vi "Error Handler.vi"(8 "error in (no error)":errorcluster) -> (0 "error out (no error)":errorcluster)   [LabVIEW 2019]
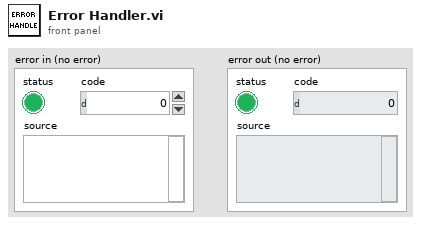
[diagram p1: front panel]
types:
  T1 = enum16{"open", "replace", "create", "open or create", "replace or create", "replace or create with confirmation"}
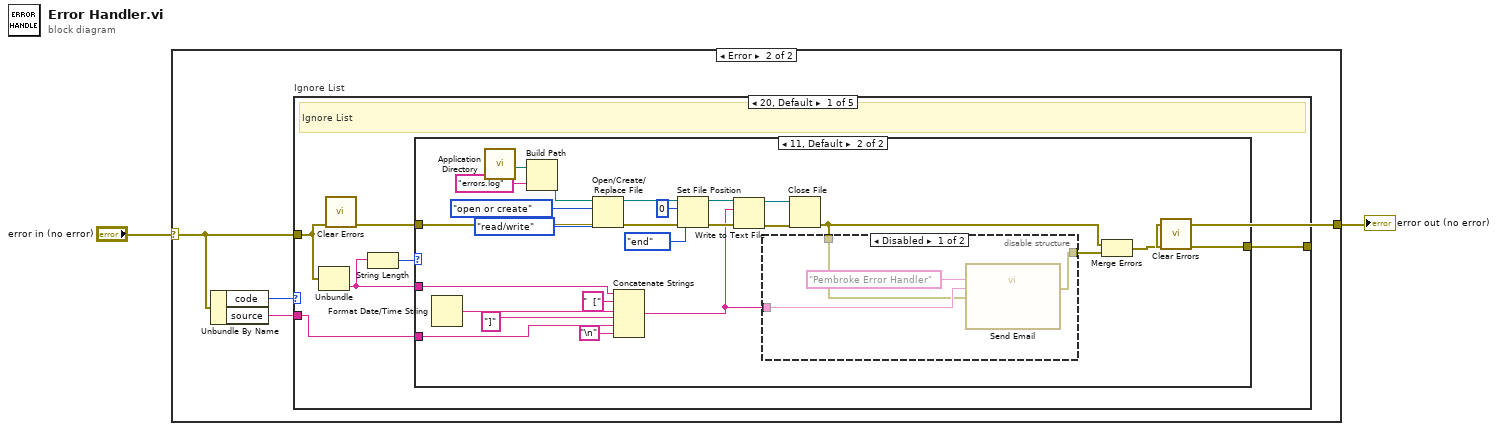
[diagram p0: block diagram]
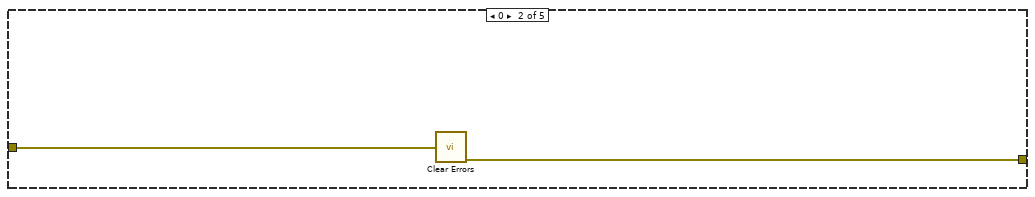
[diagram p5: hidden frame]
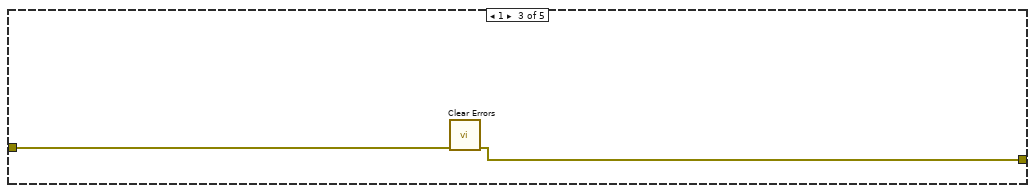
[diagram p6: hidden frame]
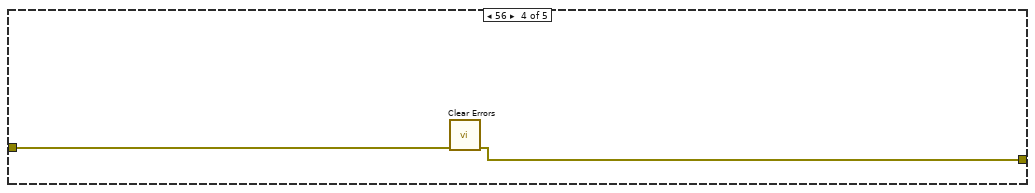
[diagram p7: hidden frame]
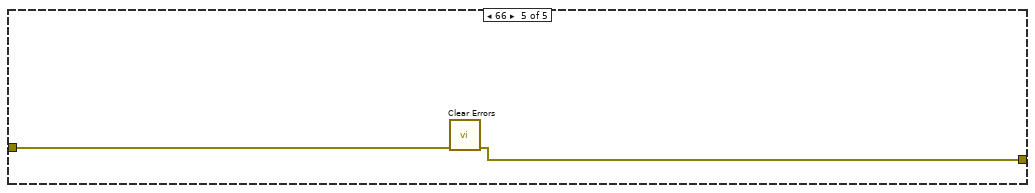
[diagram p8: hidden frame]
diagram:
  n1 = case shown="Error" "error in (no error)" {
    selector: "error in (no error)" -> [w3 w6]
    tunnel: [w3 w7] -> w2
    frame No Error {
    }
    frame Error {
      n2 = Unbundle By Name(w6) -> ("code"=w5:i32, "source"=w4:string)
      n3 = case "Ignore List" shown="20, Default" w5 {
        tunnel: w6 -> [w12 w46 w48 w50 w52]
        tunnel: [w11 w45 w47 w49 w51] -> w7
        tunnel: w4 -> [w8 _ _ _ _]
        frame 20, Default {
          # "Ignore List"
          n4 = Unbundle(w12) -> ("source"=w10:string)  [unwired: 2 out]
          n5 = call <vilib>:"Clear Errors.vi"("error in (no error)"=w12) -> ("error out"=w13:errorcluster)  [unwired: 5 in, 1 out]
          n6 = String Length(string=w10) -> (length=w9:i32)
          n7 = case shown="11, Default" w9 {
            tunnel: w13 -> [w14 w26]
            tunnel: w8 -> [_ w19]
            tunnel: [w14 w16] -> w11
            tunnel: w10 -> [_ w15]
            frame 0..10 {
            }
            frame 11, Default {
              n8 = Format Date/Time String() -> (date/time string=w23:string)  [unwired: 3 in]
              n9 = call <vilib>:"Application Directory.vi"() -> ("Application Directory"=w38:path)
              n10 = Build Path(base path=w38, name or relative path="errors.log") -> (appended path=w37:path)
              n11 = Open/Create/Replace File(file path (use dialog)=w37, error in=w26, operation (0:open)=T1."open or create", access (0:read/write)=enum16{"read/write", "read-only", "write-only"}."read/write") -> (refnum out=w32:refnum<file>, error out=w31:errorcluster)  [unwired: 2 in, 1 out]
              n12 = Concatenate Strings(w15, "  [" ("string"), w23, "]" ("string"), w19, "\n") -> (w22:string)
              n13 = Set File Position(offset (in bytes) (0)=i64 0, refnum=w32, from (0:start)=enum16{"start", "end", "current"}."end", error in=w31) -> (refnum out=w29:refnum<file>, error out=w30:errorcluster)
              n14 = Write to Text File(file (use dialog)=w29, text=w22, error in=w30) -> (refnum out=w35:refnum<file>, error out=w36:errorcluster)  [unwired: 1 in, 1 out]
              n15 = Close File(refnum=w35, error in=w36) -> (error out=w21:errorcluster)  [unwired: 1 out]
              n16 = disable-structure shown="Disabled" {
                disable-tunnel: w22 -> [w43 _]
                disable-tunnel: w21 -> [w41 w44]
                disable-tunnel: [w40 w44] -> w20
                frame Disabled {
                  n17 = call "Send Email"("error in"=w41, "Message"=w43, "Subject"="Pembroke Error Handler") -> ("error out"=w40:errorcluster)  [unwired: 8 in]
                }
                frame Enabled {
                }
              }
              n18 = Merge Errors(w21, w20) -> (w17:errorcluster)
              n19 = call <vilib>:"Clear Errors.vi"("error in (no error)"=w17) -> ("error out"=w16:errorcluster)  [unwired: 5 in, 1 out]
            }
          }
        }
        frame 0 {
          n20 = call <vilib>:"Clear Errors.vi"("error in (no error)"=w46) -> ("error out"=w45:errorcluster)  [unwired: 5 in, 1 out]
        }
        frame 1 {
          n21 = call <vilib>:"Clear Errors.vi"("error in (no error)"=w48) -> ("error out"=w47:errorcluster)  [unwired: 5 in, 1 out]
        }
        frame 56 {
          n22 = call <vilib>:"Clear Errors.vi"("error in (no error)"=w50) -> ("error out"=w49:errorcluster)  [unwired: 5 in, 1 out]
        }
        frame 66 {
          n23 = call <vilib>:"Clear Errors.vi"("error in (no error)"=w52) -> ("error out"=w51:errorcluster)  [unwired: 5 in, 1 out]
        }
      }
    }
  }
  "error out (no error)" <- w2
